vi "RenameDB.vi"(8 "error in":errorcluster, 10 "New File Name (with extension)":string, 11 "object in":refnum<class "TableLogger_Actor.lvclass">) -> (0 "error out":errorcluster, 3 "object out":refnum<class "TableLogger_Actor.lvclass">)   [LabVIEW 2014, in "TableLogger_Actor.lvlib" / "TableLogger_Actor.lvclass"]
uses:
  TableLogger_Actor.lvclass
  TableLogger_Actor.lvclass/TableLogger_Actor.ctl
panel:
  # "Connector Pane"
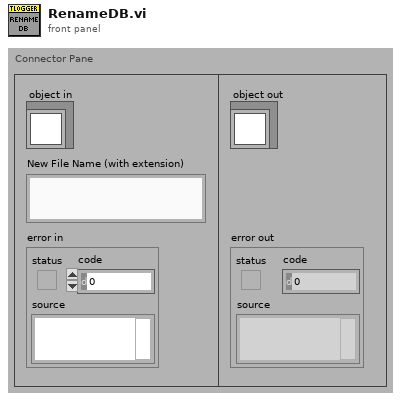
[diagram p1: front panel]
types:
  T1 = typedef "TableLogger_Actor.lvlib/TableLoggerConfig.ctl" = cluster{"TableLogger":T2, "DB File Path":path, "DB Backup Config":T3}
  T2 = typedef "TableLogger_Actor.lvlib/TableLoggerTypes.ctl" = enum16{"CSV Logger", "SQLite Logger"}
  T3 = typedef "TableLogger_Actor.lvlib/TableLoggerBackupConfig.ctl" = cluster{"Directory":path, "UTC Time Format":bool, "On Launch":bool, "Interval (Hours)":dbl, "Size Multiples (Bytes)":i32}
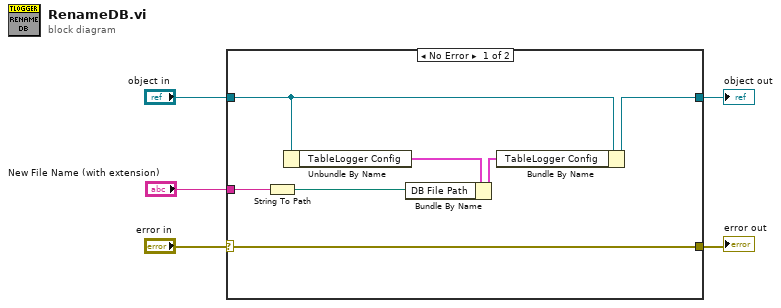
[diagram p0: block diagram]
diagram:
  n1 = case shown="No Error" "error in" {
    selector: "error in" -> [w11 w14]
    tunnel: [w11 w14] -> w4
    tunnel: [w9 w13] -> w2
    tunnel: "object in" -> [w10 w13]
    tunnel: "New File Name (with extension)" -> [w7 _]
    frame No Error {
      n2 = String To Path(string=w7) -> (path=w6:path)
      n3 = Unbundle By Name(w10) -> ("TableLogger Config"=w12:T1)
      n4 = Bundle By Name(cluster=w12, "DB File Path"=w6) -> (w8:T1)
      n5 = Bundle By Name(cluster=w10, "TableLogger Config"=w8) -> (w9:refnum<class "TableLogger_Actor.lvclass">)
    }
    frame Error {
    }
  }
  "error out" <- w4
  "object out" <- w2
